vi "Initialize.vi"(8 "error in":errorcluster, 10 "parameters":variant, 11 "PS Channel in":refnum<class "Power Supply Channel.lvclass">) -> (0 "error out":errorcluster, 2 "summary":T2[](array[typedef]), 3 "data value reference":T1)   [LabVIEW 2025, in "Power Supply.lvlib" / "Power Supply Channel.lvclass"]
doc: "This Vi initializes the data of a node its default state.\nThe object is not created inside of this ViI, beacuase it is created from a File depending on user selection.Copyright 2017 National Instruments Corporation\n\nLicensed under the Apache License, Version 2.0 (the \"License\"); you may not use this file except in compliance with the License. You may obtain a copy of the License at http://www.apache.org/licenses/LICENSE-2.0\nUnless required by applicable law or agreed to in writing, software distributed under the License is distributed on an \"AS IS\" BASIS, WITHOUT WARRANTIES OR CONDITIONS OF ANY KIND, either express or implied. See the License for the specific language governing permissions and limitations under the License."
uses:
  Power Supply Channel.lvclass
  Power Supply Channel.lvclass/Power Supply Channel.ctl
  Users/Public/Documents/Sandia National Labs/TSS Plugin/CEF.lvlibp/Node/CEF_Node.lvclass
  PS Instrument/Power Supply Instrument.lvclass
  Users/Public/Documents/Sandia National Labs/TSS Plugin/Abstract Engine.lvlibp/Plugin/Abstract/Instrument configuration/Instrument configuration.lvclass
  Users/Public/Documents/Sandia National Labs/TSS Plugin/Abstract Engine.lvlibp/Plugin/Abstract/Abstract Channel/Abstract Channel.lvclass
  PS Channel configuration/Power Supply Channel configuration.lvclass
  Users/Public/Documents/Sandia National Labs/TSS Plugin/CEF.lvlibp/Node/NodeRef.ctl
  Users/Public/Documents/Sandia National Labs/TSS Plugin/CEF.lvlibp/Node/Summary.ctl
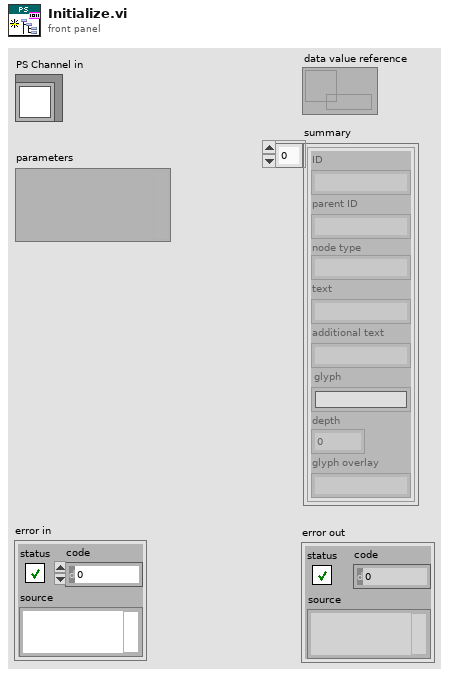
[diagram p1: front panel]
types:
  T1 = typedef "CEF.lvlibp/CEF_Node.lvclass/NodeRef.ctl" = refnum<data-value>
  T2 = typedef "CEF.lvlibp/CEF_Node.lvclass/Summary.ctl" = cluster{"ID":string, "parent ID":string, "node type":string, "text":string, "additional text":string, "glyph":string, "depth":i32, "glyph overlay":string}
  T3 = cluster{"Type":string, "Address":string, "SW Alias":string, "Description":string, "Enabled":bool}
  T4 = cluster{"Address":string, "SW Alias":string, "Enabled":bool, "Type":string, "Description":string}
  T5 = cluster{"ID":string, "parent ID":string, "node type":string, "text":string, "additional text":string, "glyph":string, "depth":i32, "glyph overlay":string}[]
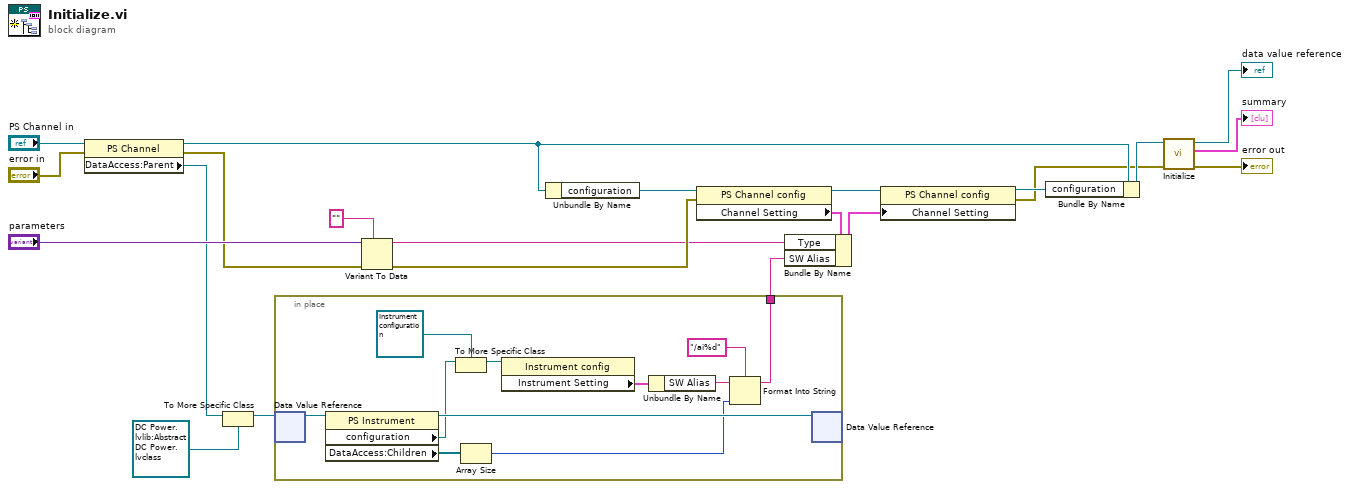
[diagram p0: block diagram]
diagram:
  n1 = property class="PS Channel"(reference="PS Channel in", error in="error in") -> (reference out=w14:refnum<class "Power Supply Channel.lvclass">, error out=w8:errorcluster, "DataAccess:Parent"=w11:refnum<data-value>)
  n2 = To More Specific Class(target class=refnum<data-value> refnum ("data value reference"), reference=w11) -> (specific class reference=w13:refnum<data-value>)  [unwired: 1 in, 1 out]
  n3 = in-place {
    in-place-border: [w31] -> w12
    n4 = in-place-dvr #1(w13) -> (w30:refnum<class "Power Supply Instrument.lvclass">)  [unwired: 1 out]
    n5 = property class="PS Instrument"(reference=w30) -> (reference out=w29:refnum<class "Power Supply Instrument.lvclass">, "configuration"=w28:refnum<class "CEF_serializable configuration.lvclass">, "DataAccess:Children"=w27:refnum<data-value>[])  [unwired: 1 in, 1 out]
    n6 = To More Specific Class(target class=refnum<class "Instrument configuration.lvclass"> refnum ("Abstract PlugIn.lvlibp:Instrument configuration"), reference=w28) -> (specific class reference=w26:refnum<class "Instrument configuration.lvclass">)  [unwired: 1 in, 1 out]
    n7 = Array Size(array=w27) -> (size(s)=w25:i32)
    n8 = property class="Instrument config"(reference=w26) -> ("Instrument Setting"=w23:T3)  [unwired: 1 in, 2 out]
    n9 = Unbundle By Name(w23) -> ("SW Alias"=w33:string)
    n10 = Format Into String(format string="/ai%d", initial string=w33, w25) -> (resulting string=w31:string)  [unwired: 1 in, 1 out]
    n11 = in-place-dvr #1(w29) -> ()  [unwired: 2 out]
  }
  n12 = Variant To Data(error in=w8, type="", Variant="parameters") -> (data=w5:string, error out=w7:errorcluster)
  n13 = Unbundle By Name(w14) -> ("configuration"=w18:refnum<class "Power Supply Channel configuration.lvclass">)
  n14 = property class="PS Channel config"(reference=w18, error in=w7) -> (reference out=w4:refnum<class "Power Supply Channel configuration.lvclass">, "Channel Setting"=w3:T4)  [unwired: 1 out]
  n15 = Bundle By Name(cluster=w3, "Type"=w5, "SW Alias"=w12) -> (w2:T4)
  n16 = property class="PS Channel config"(reference=w4, "Channel Setting"=w2) -> (reference out=w19:refnum<class "Power Supply Channel configuration.lvclass">, error out=w9:errorcluster)  [unwired: 1 in]
  n17 = Bundle By Name(cluster=w14, "configuration"=w19) -> (w16:refnum<class "Power Supply Channel.lvclass">)
  n18 = call-parent "Initialize.vi"("error in"=w9, "CEF_Serialize node in"=w16) -> ("error out"=→"error out":errorcluster, "summary"=→"summary":T5, "data value reference"=→"data value reference":refnum<data-value>)  [unwired: 7 in]
